vi "Read_Joint_States_A.vi"(4 "node":string, 5 "error in":errorcluster, 8 "Units (deg)":enum16{"Radians", "Degrees"}(ring)=enum."Degrees") -> (0 "error out":errorcluster, 1 "right Positions":dbl[](array[numeric]), 2 "left Positions":dbl[](array[numeric]), 3 "Joint States":T1(array[cluster]))   [LabVIEW 2013]
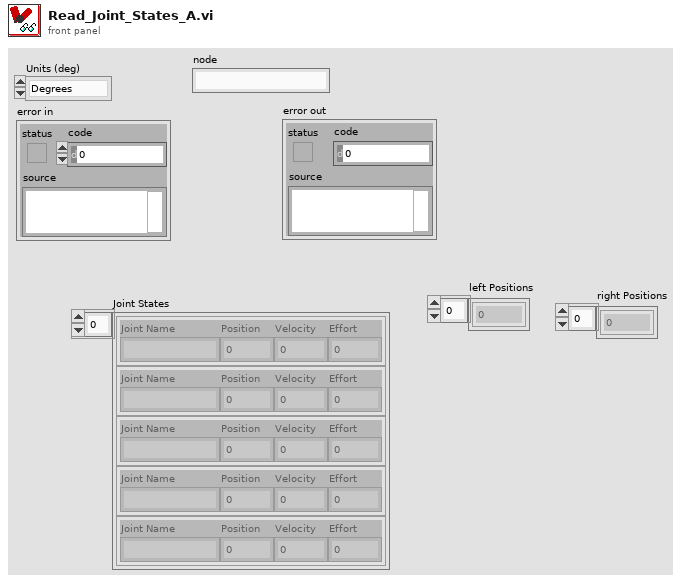
[diagram p1: front panel]
types:
  T1 = cluster{"Joint Name":string, "Position":dbl, "Velocity":dbl, "Effort":dbl}[]
  T2 = typedef "JointPositions.ctl" = cluster{"e0":dbl, "e1":dbl, "s0":dbl, "s1":dbl, "w0":dbl, "w1":dbl, "w2":dbl}
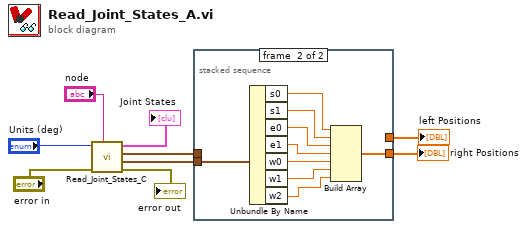
[diagram p0: block diagram]
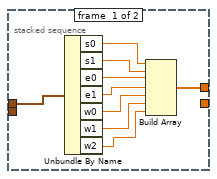
[diagram p2: hidden frame]
diagram:
  n1 = call "Read_Joint_States_C.vi"("node"="node", "error in"="error in", "Units (deg)"="Units (deg)") -> ("error out"=→"error out":errorcluster, "right Positions"=w2:T2, "left Positions"=w4:T2, "Joint States"=→"Joint States":T1)  [unwired: 2 in]
  n2 = stacked-sequence {
    tunnel: w4 -> [w18 _]
    tunnel: [w10 _] -> w3
    tunnel: w2 -> [_ w20]
    tunnel: [_ w19] -> w1
    frame #0 {
      n3 = Unbundle By Name(w18) -> ("s0"=w17:dbl, "s1"=w16:dbl, "e0"=w15:dbl, "e1"=w14:dbl, "w0"=w13:dbl, "w1"=w12:dbl, "w2"=w11:dbl)
      n4 = Build Array(w17, w16, w15, w14, w13, w12, w11) -> (w10:dbl[])
    }
    frame #1 {
      n5 = Unbundle By Name(w20) -> ("s0"=w27:dbl, "s1"=w26:dbl, "e0"=w25:dbl, "e1"=w24:dbl, "w0"=w23:dbl, "w1"=w22:dbl, "w2"=w21:dbl)
      n6 = Build Array(w27, w26, w25, w24, w23, w22, w21) -> (w19:dbl[])
    }
  }
  "left Positions" <- w3
  "right Positions" <- w1
